vi "Stack suenf.vi"() -> ()   [LabVIEW 2011]
panel:
  out "Z":dbl
  in  "Y":dbl
  in  "X":dbl
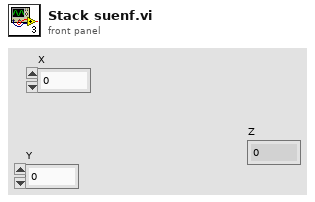
[diagram p1: front panel]
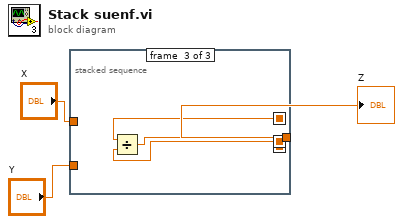
[diagram p0: block diagram]
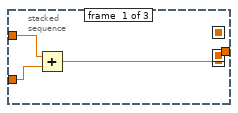
[diagram p2: hidden frame]
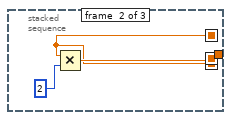
[diagram p3: hidden frame]
diagram:
  n1 = stacked-sequence {
    seq-local: [w4 _ _] -> [_ w7 _]
    seq-local: [_ w8 _] -> [_ _ w11]
    seq-local: [_ w7 _] -> [_ _ w12]
    tunnel: "X" -> [w6 _ _]
    tunnel: "Y" -> [w5 _ _]
    tunnel: [_ _ w10] -> w1
    frame #0 {
      n2 = Add(x=w6, y=w5) -> (x+y=w4:dbl)
    }
    frame #1 {
      n3 = Multiply(x=w7, y=2) -> (x*y=w8:dbl)
    }
    frame #2 {
      n4 = Divide(x=w12, y=w11) -> (x/y=w10:dbl)
    }
  }
  "Z" <- w1
